vi "CalculateSpeedWithCache.vi"(8 "error in (no error)":errorcluster, 9 "pulse cache":T1, 11 "Pulse Positions":dbl[](array[numeric])) -> (0 "error out":errorcluster, 2 "Speed (RPM)":dbl)   [LabVIEW 2017, in "AnalysisHelper.lvlib"]
uses:
  <vilib>/addons/InsightCM/Utilities/Analysis/Shared/AnalysisHelper.lvlib
  <vilib>/addons/InsightCM/Utilities/Analysis/Shared/controls/SpeedCache.ctl
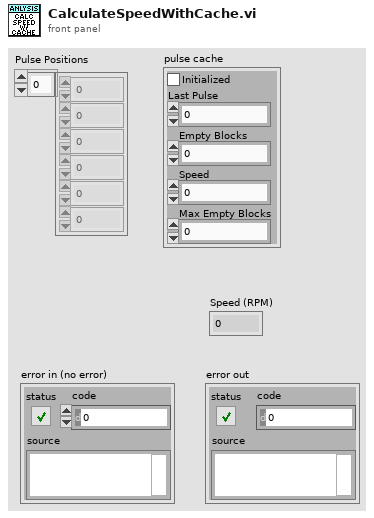
[diagram p1: front panel]
types:
  T1 = typedef "AnalysisHelper.lvlib/SpeedCache.ctl" = cluster{"Initialized":bool, "Last Pulse":dbl, "Empty Blocks":i32, "Speed":dbl, "Max Empty Blocks":i32}
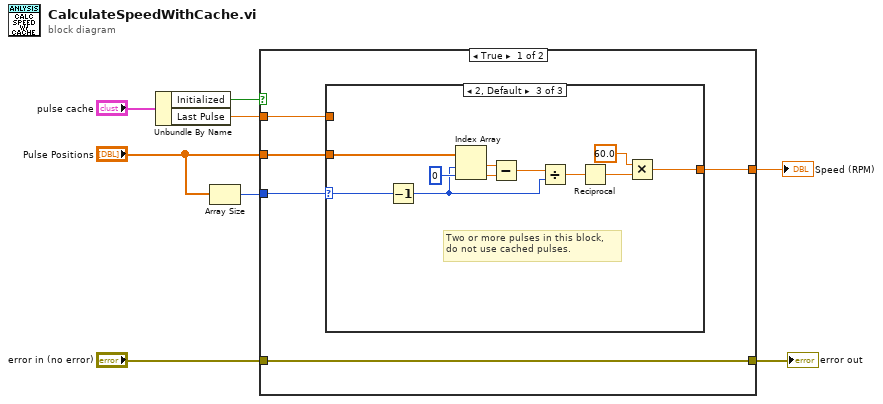
[diagram p0: block diagram]
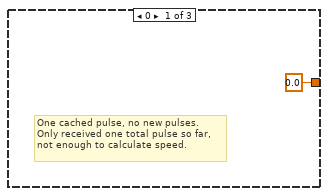
[diagram p2: hidden frame]
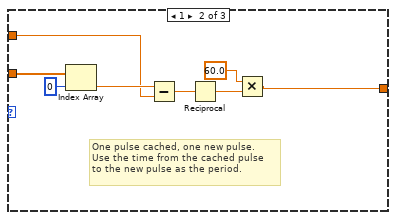
[diagram p3: hidden frame]
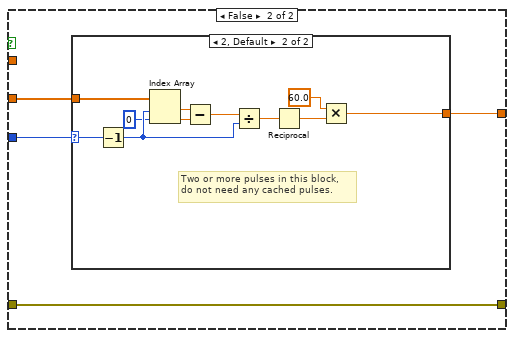
[diagram p4: hidden frame]
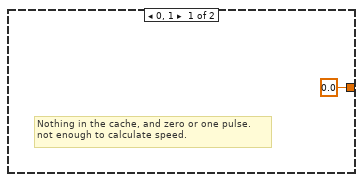
[diagram p5: hidden frame]
diagram:
  n1 = Unbundle By Name("pulse cache") -> ("Initialized"=w1:bool, "Last Pulse"=w4:dbl)
  n2 = Array Size(array="Pulse Positions") -> (size(s)=w2:i32)
  n3 = case shown="True" w1 {
    tunnel: [w12 w37] -> w6
    tunnel: "Pulse Positions" -> [w11 w35]
    tunnel: [w13 w36] -> w8
    tunnel: "error in (no error)" -> [w13 w36]
    tunnel: w4 -> [w10 _]
    tunnel: w2 -> [w9 w34]
    frame True {
      n4 = case shown="2, Default" w9 {
        selector: w9 -> [_ _ w25]
        tunnel: [0.0 w15 w26] -> w12
        tunnel: w11 -> [_ w22 w24]
        tunnel: w10 -> [_ w19 _]
        frame 0 {
          # "One cached pulse, no new pulses.\nOnly received one total pulse so far,\nnot enough to calculate speed."
        }
        frame 1 {
          # "One pulse cached, one new pulse.\nUse the time from the cached pulse\nto the new pulse as the period."
          n5 = Index Array(array=w22, index=0) -> (element=w20:dbl)
          n6 = Subtract(x=w20, y=w19) -> (x-y=w16:dbl)
          n7 = Reciprocal(x=w16) -> (1/x=w17:dbl)
          n8 = Multiply(x=sgl 60.0, y=w17) -> (x*y=w15:dbl)
        }
        frame 2, Default {
          # "Two or more pulses in this block,\ndo not use cached pulses."
          n9 = Decrement(x=w25) -> (x-1=w23:i32)
          n10 = Index Array(array=w24, index #1=w23, index #2=0 ("index")) -> (element #1=w31:dbl, element #2=w29:dbl)
          n11 = Subtract(x=w31, y=w29) -> (x-y=w32:dbl)
          n12 = Divide(x=w32, y=w23) -> (x/y=w28:dbl)
          n13 = Reciprocal(x=w28) -> (1/x=w27:dbl)
          n14 = Multiply(x=sgl 60.0, y=w27) -> (x*y=w26:dbl)
        }
      }
    }
    frame False {
      n15 = case shown="2, Default" w34 {
        selector: w34 -> [_ w39]
        tunnel: [0.0 w49] -> w37
        tunnel: w35 -> [_ w40]
        frame 0, 1 {
          # "Nothing in the cache, and zero or one pulse.\nnot enough to calculate speed."
        }
        frame 2, Default {
          # "Two or more pulses in this block,\ndo not need any cached pulses."
          n16 = Decrement(x=w39) -> (x-1=w47:i32)
          n17 = Index Array(array=w40, index #1=w47, index #2=0 ("index")) -> (element #1=w45:dbl, element #2=w43:dbl)
          n18 = Subtract(x=w45, y=w43) -> (x-y=w46:dbl)
          n19 = Divide(x=w46, y=w47) -> (x/y=w42:dbl)
          n20 = Reciprocal(x=w42) -> (1/x=w41:dbl)
          n21 = Multiply(x=sgl 60.0, y=w41) -> (x*y=w49:dbl)
        }
      }
    }
  }
  "Speed (RPM)" <- w6
  "error out" <- w8
